vi "终止项.vi"(1 "结果":i32[][](array[numeric]), 2 "检索":i32[][](array[numeric])) -> (0 "数值":i32)   [LabVIEW 2014]
panel:
  out "结果 2":i32[][](array[numeric])
  out "检索 2":i32[][](array[numeric])
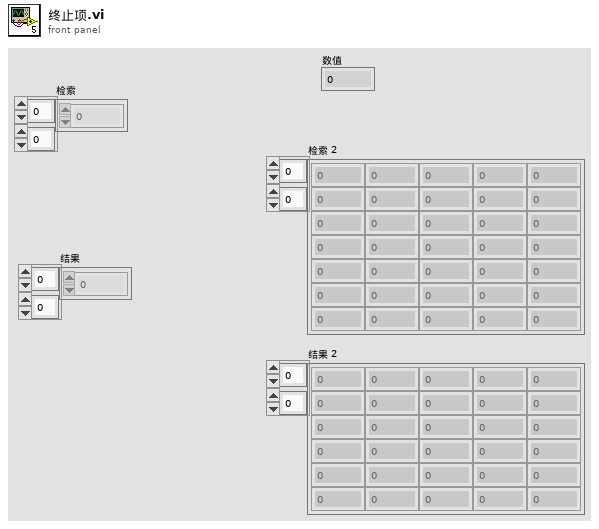
[diagram p1: front panel]
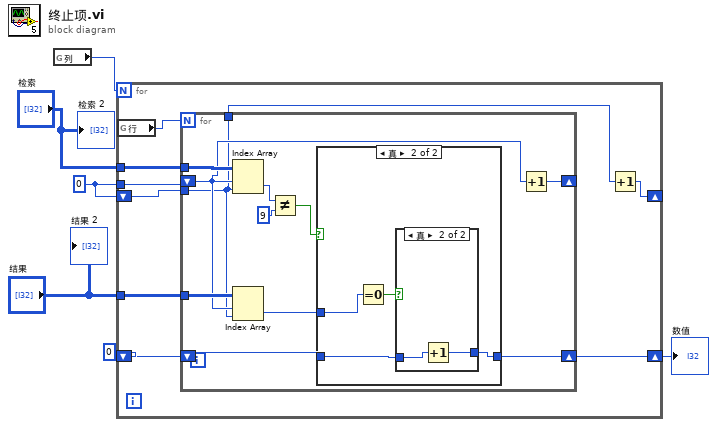
[diagram p0: block diagram]
diagram:
  w3 = 0
  n1 = global read "全局 1.vi" "列"() -> (w1:i32)
  n2 = for {
    N: w1 -> [_]
    tunnel: "检索" -> [w15]
    tunnel: "结果" -> [w14]
    shift-right: [w13] -> w2
    shift-left: 0 -> [w12]
    tunnel: w3 -> [w10]
    shift-right: [w9] -> _
    shift-left: w3 -> [w8]
    n3 = global read "全局 1.vi" "行"() -> (w7:i32)
    n4 = for {
      N: w7 -> [_]
      tunnel: w15 -> [w26]
      tunnel: w8 -> [w16]
      tunnel: w14 -> [w22]
      shift-right: [w20] -> w13
      shift-left: w12 -> [w19]
      shift-right: [w18] -> _
      shift-left: w10 -> [w17]
      tunnel: [w16] -> w11
      n5 = Index Array(array=w26, index (row)=w17, index (col)=w16) -> (element=w25:i32)
      n6 = Index Array(array=w22, index (row)=w17, index (col)=w16) -> (element=w21:i32)
      n7 = Not Equal?(x=w25, y=9) -> (x != y?=w23:bool)
      n8 = case shown="真" w23 {
        tunnel: w21 -> [_ w31]
        tunnel: w19 -> [w27 w30]
        tunnel: [w27 w29] -> w20
        frame False {
        }
        frame True {
          n9 = Equal To 0?(x=w31) -> (x = 0?=w28:bool)
          n10 = case shown="真" w28 {
            tunnel: w30 -> [w32 w34]
            tunnel: [w32 w33] -> w29
            frame False {
            }
            frame True {
              n11 = Increment(x=w34) -> (x+1=w33:i32)
            }
          }
        }
      }
      n12 = Increment(x=w17) -> (x+1=w18:i32)
    }
    n13 = Increment(x=w11) -> (x+1=w9:i32)
  }
  "数值" <- w2
  "检索 2" <- "检索"
  "结果 2" <- "结果"
